vi "SRX_Read Errors and Faults.vi"(8 "Error":errorcluster, 11 "PhoenixMotorControlDevRef":T2={"DeviceStatus"={"status"=FALSE, "code"=0, "source"=""}, "Type"=enum."PWM", "PWM"={"PWM Channel"=enum."Invalid", "DeadBand"={"Name"="", "maxPositivePwm"=0, "minPositivePwm"=0, "centerPwm"=0, "maxNegativePwm"=0, "minNegativePwm"=0, "angularRange"=0}}, "CAN"={"Device Number"=0, "SetOutput VI Ref"=variant(enum8{"Percent VBus", "Current", "Speed", "Position", "Voltage"} enum."Percent VBus"), "GetOutput VI Ref"=variant(refnum<k1> refnum), "Enable VI Ref"=variant(dbl 12.0), "Disable VI Ref"=variant(enum8{"Percent VBus", "Speed", "Position", "Slave", "Unchanged / Invalid", "Voltage Compensation", "Current", "Motion Profile"} enum."Percent VBus"), "Data"=variant}, "Invert"=FALSE, "DIO PWM"={"PWM \"Enable\" Channel"=enum."Invalid", "DIOChannel"=enum."Invalid", "PWM Rate"=0.0}}) -> (0 "Error Out":errorcluster, 2 "Last Error Code Out":i32, 3 "Faults Out":T1)   [LabVIEW 2017]
uses:
  <vilib>/Rock Robotics/WPI/MotorControl/WPI_MotorControlDeviceRef.ctl
  <vilib>/Rock Robotics/WPI/MotorControl/WPI_MotorControlType.ctl
  <vilib>/Rock Robotics/SystemInterfaces/DIO/FPGA_DIOPWMChannel.ctl
  <vilib>/Rock Robotics/WPI/PWM/WPI_PWMDeadband.ctl
  <vilib>/Rock Robotics/SystemInterfaces/DIO/FPGA_DIOChannel.ctl
  TypeDefs SRX/Cluster_SRX_Faults.ctl
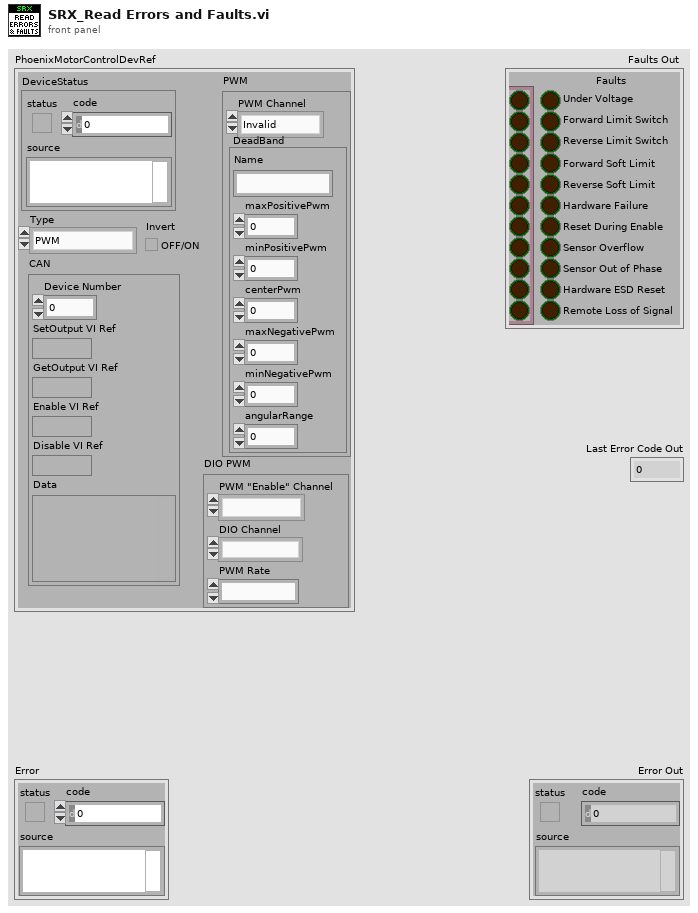
[diagram p1: front panel]
types:
  T1 = typedef "Cluster_SRX_Faults.ctl" = cluster{"Sticky":cluster{"Under Voltage":bool, "Forward Limit Switch":bool, "Reverse Limit Switch":bool, "Forward Soft Limit":bool, "Reverse Soft Limit":bool, "Hardware Failure":bool, "Reset During Enable":bool, "Sensor Overflow":bool, "Sensor Out of Phase":bool, "Hardware ESD Reset":bool, "Remote Loss of Signal":bool}, "Faults":cluster{"Under Voltage":bool, "Forward Limit Switch":bool, "Reverse Limit Switch":bool, "Forward Soft Limit":bool, "Reverse Soft Limit":bool, "Hardware Failure":bool, "Reset During Enable":bool, "Sensor Overflow":bool, "Sensor Out of Phase":bool, "Hardware ESD Reset":bool, "Remote Loss of Signal":bool}}
  T2 = typedef "WPI_MotorControlDeviceRef.ctl" = cluster{"DeviceStatus":errorcluster, "Type":T3, "PWM":cluster{"PWM Channel":T4, "DeadBand":T5}, "CAN":cluster{"Device Number":u8, "SetOutput VI Ref":variant, "GetOutput VI Ref":variant, "Enable VI Ref":variant, "Disable VI Ref":variant, "Data":variant}, "Invert":bool, "DIO PWM":cluster{"PWM \"Enable\" Channel":T4, "DIOChannel":T6, "PWM Rate":dbl}}
  T3 = typedef "WPI_MotorControlType.ctl" = enum16{"PWM", "CAN", "DIO PWM"}
  T4 = typedef "FPGA_DIOPWMChannel.ctl" = enum8{"PWM 0", "PWM 1", "PWM 2", "PWM 3", "PWM 4", "PWM 5", "PWM 6", "PWM 7", "PWM 8", "PWM 9", "PWM MXP 0", "PWM MXP 1", "PWM MXP 2", "PWM MXP 3", "PWM MXP 4", "PWM MXP 5", "PWM MXP 6", "PWM MXP 7", "PWM MXP 8", "PWM MXP 9", "Invalid"}
  T5 = typedef "WPI_PWMDeadband.ctl" = cluster{"Name":string, "maxPositivePwm":i32, "minPositivePwm":i32, "centerPwm":i32, "maxNegativePwm":i32, "minNegativePwm":i32, "angularRange":u16}
  T6 = typedef "FPGA_DIOChannel.ctl" = enum8{"DIO 0", "DIO 1", "DIO 2", "DIO 3", "DIO 4", "DIO 5", "DIO 6", "DIO 7", "DIO 8", "DIO 9", "DIO MXP 0", "DIO MXP 1", "DIO MXP 2", "DIO MXP 3", "DIO MXP 4", "DIO MXP 5", "DIO MXP 6", "DIO MXP 7", "DIO MXP 8", "DIO MXP 9", "DIO MXP 10", "DIO MXP 11", "DIO MXP 12", "DIO MXP 13", "DIO MXP 14", "DIO MXP 15", "SPI Port CS1", "SPI Port CS2", "SPI Port CS3", "SPI Port MISO", "SPI Port MOSI", "Invalid"}
  T7 = cluster{"Under Voltage":bool, "Forward Limit Switch":bool, "Reverse Limit Switch":bool, "Forward Soft Limit":bool, "Reverse Soft Limit":bool, "Hardware Failure":bool, "Reset During Enable":bool, "Sensor Overflow":bool, "Sensor Out of Phase":bool, "Hardware ESD Reset":bool, "Remote Loss of Signal":bool}
  T8 = cluster{"Under Voltage":bool, "Forward Limit Switch":bool, "Reverse Limit Switch":bool, "Forward Soft Limit":bool, "Reverse Soft Limit":bool, "Reset During Enable":bool, "Sensor Overflow":bool, "Sensor Out of Phase":bool, "Hardware ESD Reset":bool, "Remote Loss of Signal":bool}
  T9 = cluster{"Sticky Faults Out[0]":bool, "Sticky Faults Out[1]":bool, "Sticky Faults Out[2]":bool, "Sticky Faults Out[3]":bool, "Sticky Faults Out[4]":bool, "Sticky Faults Out[5]":bool, "Sticky Faults Out[6]":bool, "Sticky Faults Out[7]":bool, "Sticky Faults Out[8]":bool, "Sticky Faults Out[9]":bool, "Sticky Faults Out[10]":bool}
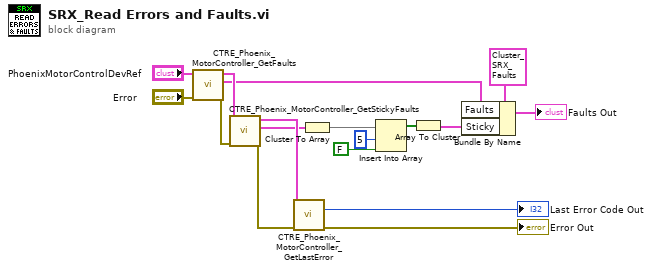
[diagram p0: block diagram]
diagram:
  n1 = call "CTRE_Phoenix_MotorController_GetFaults.vi"("Error"="Error", "PhoenixMotorControlDevRef"="PhoenixMotorControlDevRef") -> ("Error Out"=w2:errorcluster, "Faults Out"=w9:T7, "PhoenixMotorControlDevRef Out"=w14:T2)  [unwired: 7 in]
  n2 = call "CTRE_Phoenix_MotorController_GetStickyFaults.vi"("Error"=w2, "PhoenixMotorControlDevRef"=w14) -> ("Error Out"=w1:errorcluster, "Sticky Faults Out"=w8:T8, "PhoenixMotorControlDevRef Out"=w13:T2)  [unwired: 7 in]
  n3 = call "CTRE_Phoenix_MotorController_GetLastError.vi"("PhoenixMotorControlDevRef"=w13, "error in"=w1) -> ("Last Error Code"=→"Last Error Code Out":i32, "error out"=→"Error Out":errorcluster)  [unwired: 11 in, 1 out]
  n4 = Cluster To Array(cluster=w8) -> (array=w7:bool[])
  n5 = Insert Into Array(array=w7, index=5, new element=FALSE ("new element/subarray")) -> (w4:bool[])
  n6 = Array To Cluster(array=w4) -> (cluster=w3:T9)
  n7 = Bundle By Name(cluster=T1 {"Sticky"={"Under Voltage"=FALSE, "Forward Limit Switch"=FALSE, "Reverse Limit Switch"=FALSE, "Forward Soft Limit"=FALSE, "Reverse Soft Limit"=FALSE, "Hardware Failure"=FALSE, "Reset During Enable"=FALSE, "Sensor Overflow"=FALSE, "Sensor Out of Phase"=FALSE, "Hardware ESD Reset"=FALSE, "Remote Loss of Signal"=FALSE}, "Faults"={"Under Voltage"=FALSE, "Forward Limit Switch"=FALSE, "Reverse Limit Switch"=FALSE, "Forward Soft Limit"=FALSE, "Reverse Soft Limit"=FALSE, "Hardware Failure"=FALSE, "Reset During Enable"=FALSE, "Sensor Overflow"=FALSE, "Sensor Out of Phase"=FALSE, "Hardware ESD Reset"=FALSE, "Remote Loss of Signal"=FALSE}} ("Faults Out"), "Faults"=w9, "Sticky"=w3) -> (→"Faults Out":T1)
